vi "TestStreamToDisk_ValueOK.vi"(8 "error in (no error)":errorcluster, 11 "TestCase in":refnum<class "TestTransport.lvclass">) -> (0 "error out":errorcluster, 3 "TestCase out":refnum<class "TestTransport.lvclass">)   [LabVIEW 2015, in "TestTransport.lvclass"]
uses:
  TestTransport.lvclass
  <vilib>/Utility/sysdir.llb/System Directory Type.ctl
  Framework/Transport/StreamToDisk/StreamToDisk.lvclass
panel:
  out "appended path":path
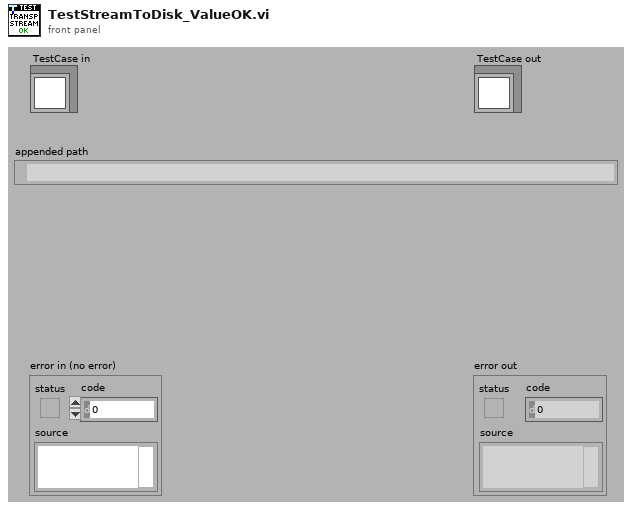
[diagram p1: front panel]
types:
  T1 = typedef "System Directory Type.ctl" = i32
  T2 = enum16{"open", "open or create", "create or replace", "create", "open (read-only)"}
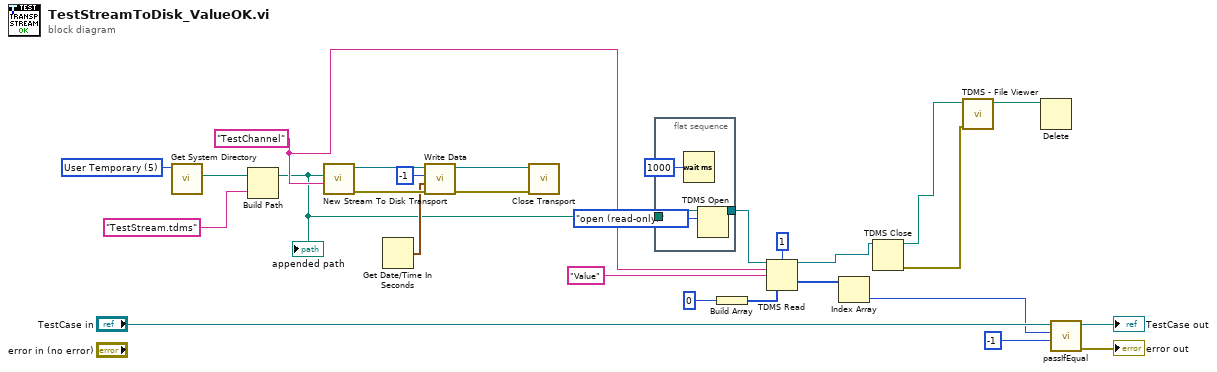
[diagram p0: block diagram]
diagram:
  w14 = "TestChannel" ("Channel Name")
  w20 = T1 5 items=["User Home"=0, "User Desktop"=1, "User Documents"=2, "User Application Data"=3, "User Preferences"=4, "User Temporary"=5, "Public Documents"=6, "Public Application Data"=7, "Public Preferences"=8, "Public Cache"=13, "System Core Libraries"=9, "System Installed Libraries"=10, "Application Files"=11, "Boot Volume Root"=12] ("system directory type")
  n1 = call <vilib>:"Get System Directory.vi"("system directory type"=w20) -> ("system directory"=w19:path)  [unwired: 10 in]
  n2 = Build Path(base path=w19, name or relative path="TestStream.tdms") -> (appended path=w11:path)
  "appended path" <- w11
  n3 = call "New Stream To Disk Transport.vi"("Channel Name"=w14, "File Path"=w11) -> ("error out"=w21:errorcluster, "StreamToDisk Out"=w22:refnum<class "StreamToDisk.lvclass">)  [unwired: 8 in]
  n4 = Get Date/Time In Seconds() -> (seconds since 1Jan1904=w12:timestamp)
  n5 = call-dynamic "Write Data.vi"("error in (no error)"=w21, "Publication Time"=w12, "Value"=-1, "StreamToDisk In"=w22) -> ("error out"=w16:errorcluster, "StreamToDisk Out"=w17:refnum<class "StreamToDisk.lvclass">)  [unwired: 6 in]
  n6 = call-dynamic "Close Transport.vi"("error in (no error)"=w16, "StreamToDisk in"=w17) -> ()  [unwired: 9 in, 1 out]
  n7 = flat-sequence {
    tunnel: w11 -> [w30]
    tunnel: [w29] -> w10
    frame #0 {
      n8 = Wait (ms)(milliseconds to wait=u32 1000) -> ()  [unwired: 1 out]
      n9 = TDMS Open(10:T2."open (read-only)" ("operation (0:open)"), 11:w30) -> (3:w29:refnum<k34>)  [unwired: 5 in, 1 out]
    }
  }
  n10 = Build Array(0) -> (w6:i32[])
  n11 = TDMS Read(0:w10, 2:i64 1 ("count (-1: all)"), 5:w14, 7:"Value" ("channel name(s) in"), 12:w6) -> (4:w5:refnum<k34>, 10:w3:i32[])  [unwired: 3 in, 4 out]
  n12 = Index Array(array=w3) -> (element=w2:i32)  [unwired: 1 in]
  n13 = TDMS Close(11:w5) -> (0:w1:errorcluster, 3:w4:path)  [unwired: 1 in]
  n14 = call <vilib>:"TDMS - File Viewer.vi"("error in (no error)"=w1, "file path"=w4) -> ("file path out"=w15:path)  [unwired: 4 in, 1 out]
  n15 = Delete(path (use dialog)=w15) -> ()  [unwired: 4 in, 3 out]
  n16 = call-dynamic "passIfEqual.vi"("y"=-1, "x"=w2, "TestCase in"="TestCase in") -> ("error out"=→"error out":errorcluster, "TestCase out"=→"TestCase out":refnum<class "TestTransport.lvclass">)  [unwired: 7 in]
